vi "Get Tasks.vi"(8 "error in (no error)":errorcluster, 11 "HAL GOOP4:Series Base in":refnum<class "Series Base.lvclass">) -> (0 "error out":errorcluster, 2 "Tasks":map{string, refnum<class "Task Base.lvclass">}(c390), 3 "HAL GOOP4:Series Base out":refnum<class "Series Base.lvclass">)   [LabVIEW 2023, in "HAL GOOP4.lvlib" / "Series Base.lvclass"]
uses:
  Series Base.lvclass
  Task Base/Task Base.lvclass
  Series Base.lvclass/Series Base.ctl
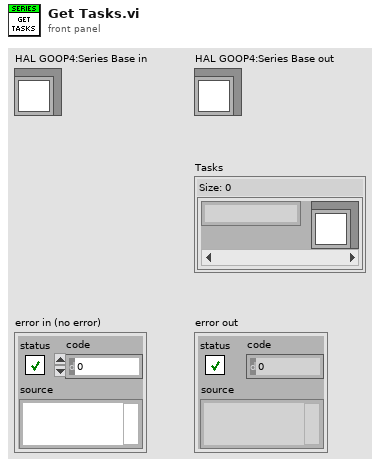
[diagram p1: front panel]
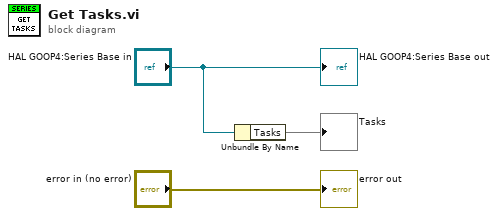
[diagram p0: block diagram]
diagram:
  n1 = Unbundle By Name("HAL GOOP4:Series Base in") -> ("Tasks"=→"Tasks":map{string, refnum<class "Task Base.lvclass">})
  "error out" <- "error in (no error)"
  "HAL GOOP4:Series Base out" <- "HAL GOOP4:Series Base in"
